vi "Ev Generate.vi"(8 "error in (no error)":errorcluster, 11 "Pic Json Generator in":refnum<class "Pic Json Generator.lvclass">) -> (0 "error out":errorcluster, 3 "Pic Json Generator out":refnum<class "Pic Json Generator.lvclass">)   [LabVIEW 2018, in "Pic Json Generator.lvlib" / "Pic Json Generator.lvclass"]
uses:
  Pic Json Generator.lvclass
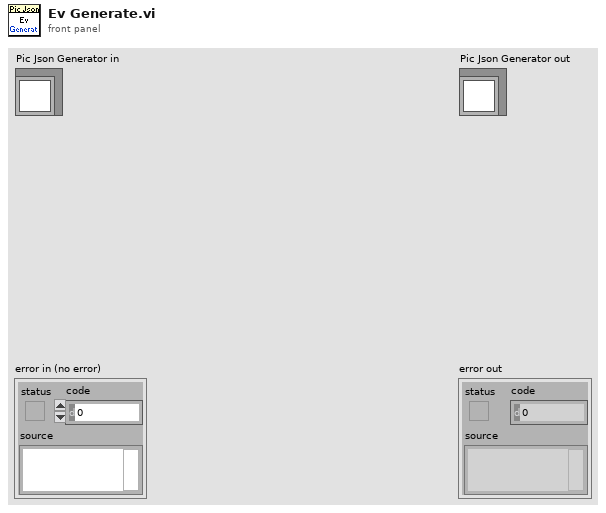
[diagram p1: front panel]
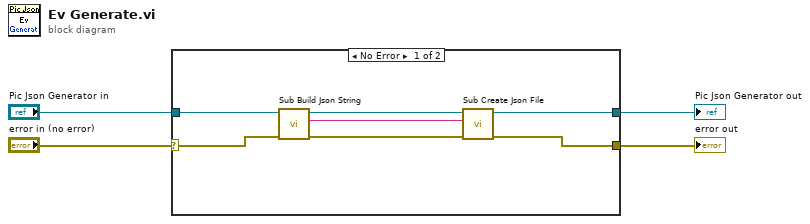
[diagram p0: block diagram]
diagram:
  n1 = case shown="No Error" "error in (no error)" {
    selector: "error in (no error)" -> [w10 w12]
    tunnel: "Pic Json Generator in" -> [w11 w13]
    tunnel: [w7 w13] -> w2
    tunnel: [w6 w12] -> w1
    frame No Error {
      n2 = call "Sub Build Json String.vi"("error in (no error)"=w10, "Pic Json Generator in"=w11) -> ("error out"=w8:errorcluster, "Json String"=w5:string, "Pic Json Generator out"=w9:refnum<class "Pic Json Generator.lvclass">)  [unwired: 7 in]
      n3 = call "Sub Create Json File.vi"("error in (no error)"=w8, "Json String"=w5, "Pic Json Generator in"=w9) -> ("error out"=w6:errorcluster, "Pic Json Generator out"=w7:refnum<class "Pic Json Generator.lvclass">)  [unwired: 7 in]
    }
    frame Error {
    }
  }
  "error out" <- w1
  "Pic Json Generator out" <- w2
